vi "-Parse_Query.vi"(8 "error in (no error)":errorcluster, 10 "Query In":string, 11 "Postgres Connector In":refnum<class "Postgres Connector.lvclass">) -> (0 "error out":errorcluster, 3 "Postgres Connector Out":refnum<class "Postgres Connector.lvclass">)   [LabVIEW 2020, in "Postgres Connector.lvclass"]
doc: "This VI build the query with the prefix and suffix"
uses:
  Postgres Connector.lvclass
  Postgres Connector.lvclass/Postgres Connector.ctl
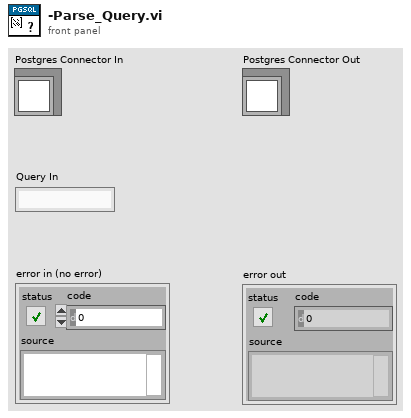
[diagram p1: front panel]
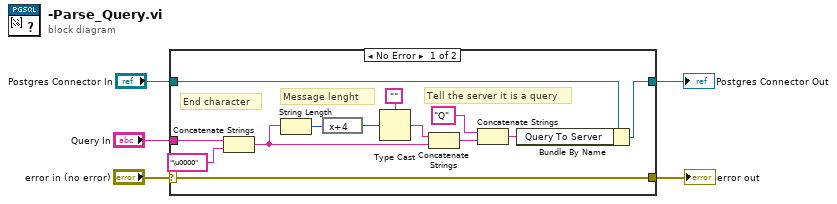
[diagram p0: block diagram]
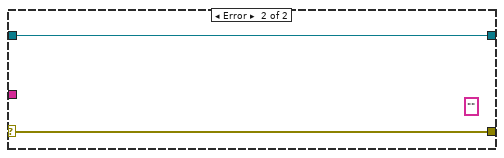
[diagram p2: hidden frame]
diagram:
  n1 = case shown="No Error" "error in (no error)" {
    selector: "error in (no error)" -> [w11 w20]
    tunnel: [w11 w20] -> w4
    tunnel: "Query In" -> [w14 _]
    tunnel: "Postgres Connector In" -> [w10 w19]
    tunnel: [w9 w19] -> w1
    frame No Error {
      # "Message lenght"
      # "Tell the server it is a query"
      # "End character"
      n2 = Concatenate Strings(w14, "\u0000") -> (w12:string)
      n3 = String Length(string=w12) -> (length=w7:i32)
      n4 = expression code="x+4"(w7) -> (w6:i32)
      n5 = Type Cast(type="", x=w6) -> (*(type *) &x=w17:string)
      n6 = Concatenate Strings(w17, w12) -> (w15:string)
      n7 = Concatenate Strings("Q", w15) -> (w8:string)
      n8 = Bundle By Name(cluster=w10, "Query To Server"=w8) -> (w9:refnum<class "Postgres Connector.lvclass">)
    }
    frame Error {
      (unwired) ""
    }
  }
  "error out" <- w4
  "Postgres Connector Out" <- w1
